vi "VectorDrive.vi"(9 "RightMotorInput":dbl, 10 "LeftMotorInput":dbl) -> (1 "RightMotorOutput":dbl, 2 "LeftMotorOutput":dbl)   [LabVIEW 2015]
uses:
  <vilib>/addons/control/pid/pid.llb/PID (DBL).vi
  navx-mxp/labview/navX Library v2/navX Library v2.lvlib
  <vilib>/addons/control/pid/NI_PID_pid.lvlib
panel:
  in  "PID gains":T1={"proportional gain (Kc)"=12.0, "integral time (Ti, min)"=0.0, "derivative time (Td, min)"=0.0015}
  in  "setpoint":dbl format="%.2f"
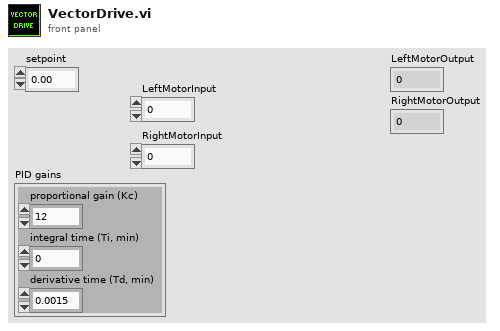
[diagram p1: front panel]
types:
  T1 = cluster{"proportional gain (Kc)":dbl, "integral time (Ti, min)":dbl, "derivative time (Td, min)":dbl}
  T2 = typedef "navX Library v2.lvlib/Z900_navX_DeviceTypeDef.ctl" = cluster{"Interface":cluster{"Protocol":T3, "Update Rate (4Hz-60Hz)":u8, "navX Open TypeDef":variant}, "Notify Packet":refnum<notifier>, "Loop VI Refnum":refnum<vi>, "Ready to Close Occurrence Refnum":refnum<k4>}
  T3 = typedef "navX Library v2.lvlib/Z900_navX_ProtocolTypeDef.ctl" = enum16{"SERIAL", "I2C", "SPI"}
  T4 = cluster{"Yaw":dbl, "Roll":dbl, "Pitch":dbl, "Heading":dbl, "Fused Heading":dbl}
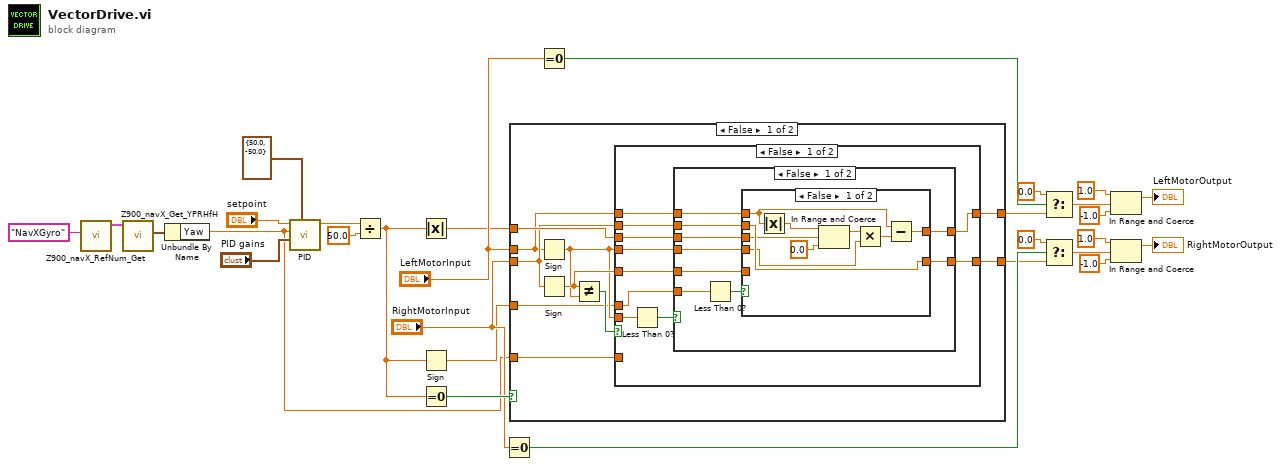
[diagram p0: block diagram]
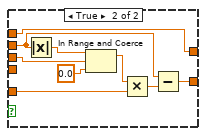
[diagram p2: hidden frame]
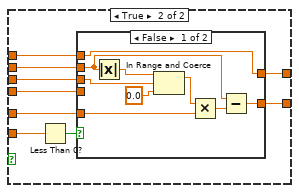
[diagram p3: hidden frame]
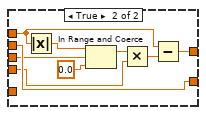
[diagram p4: hidden frame]
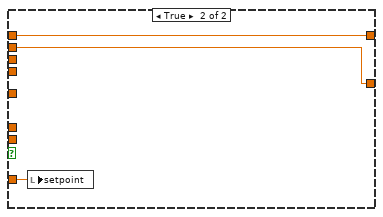
[diagram p5: hidden frame]
diagram:
  n1 = call "Z900_navX_RefNum_Get.vi"("refnum name"="NavXGyro") -> ("navX Device"=w28:T2)  [unwired: 9 in, 1 out]
  n2 = call "Z900_navX_Get_YPRHfH.vi"("navX Device"=w28) -> ("YRPHfH"=w27:T4)  [unwired: 7 in, 3 out]
  n3 = Unbundle By Name(w27) -> ("Yaw"=w12:dbl)
  n4 = call-poly <vilib>:"PID.vi"("output range"=cluster{"output high":dbl, "output low":dbl} {"output high"=50.0, "output low"=-50.0}, "PID gains"="PID gains", "process variable"=w12, "setpoint"="setpoint") -> ("output"=w1:dbl)  [unwired: 6 in, 1 out]
  n5 = Divide(x=w1, y=50.0) -> (x/y=w11:dbl)
  n6 = Absolute Value(x=w11) -> (abs(x)=w13:dbl)
  n7 = Sign(1:w11) -> (0:w10:dbl)
  n8 = Equal To 0?(x=w11) -> (x = 0?=w22:bool)
  n9 = Equal To 0?(x="RightMotorInput") -> (x = 0?=w17:bool)
  n10 = case shown="False" w22 {
    tunnel: "LeftMotorInput" -> [w34 w108]
    tunnel: "RightMotorInput" -> [w37 w107]
    tunnel: [w33 w108] -> w18
    tunnel: [w35 w107] -> w15
    tunnel: w13 -> [w38 _]
    tunnel: w12 -> [w31 _]
    tunnel: w10 -> [w30 _]
    frame False {
      n11 = Sign(1:w34) -> (0:w32:dbl)
      n12 = Sign(1:w37) -> (0:w36:dbl)
      n13 = Not Equal?(x=w36, y=w32) -> (x != y?=w39:bool)
      n14 = case shown="False" w39 {
        tunnel: w32 -> [w48 _]
        tunnel: w38 -> [w47 _]
        tunnel: w37 -> [w46 w105]
        tunnel: w36 -> [w45 _]
        tunnel: [w44 w105] -> w35
        tunnel: w34 -> [w43 w106]
        tunnel: [w42 w106] -> w33
        tunnel: w32 -> [w41 _]
        tunnel: w31 -> [_ w104]
        tunnel: w30 -> [w40 _]
        frame False {
          n15 = Less Than 0?(x=w48) -> (x < 0?=w49:bool)
          n16 = case shown="False" w49 {
            tunnel: w47 -> [w51 w80]
            tunnel: w46 -> [w55 w81]
            tunnel: w45 -> [w50 w82]
            tunnel: [w54 w77] -> w44
            tunnel: w43 -> [w53 w83]
            tunnel: [w56 w78] -> w42
            tunnel: w41 -> [w52 w79]
            tunnel: w40 -> [w58 w84]
            frame False {
              n17 = Less Than 0?(x=w58) -> (x < 0?=w57:bool)
              n18 = case shown="False" w57 {
                tunnel: [w67 w68] -> w56
                tunnel: [w66 w69] -> w54
                tunnel: w55 -> [w66 w71]
                tunnel: w53 -> [w60 w68]
                tunnel: w52 -> [w63 _]
                tunnel: w51 -> [w62 w70]
                tunnel: w50 -> [_ w72]
                frame False {
                  n19 = Absolute Value(x=w60) -> (abs(x)=w59:dbl)
                  n20 = In Range and Coerce(upper limit=w59, x=w62, lower limit=0.0) -> (coerced(x)=w64:dbl)  [unwired: 1 out]
                  n21 = Multiply(x=w64, y=w63) -> (x*y=w65:dbl)
                  n22 = Subtract(x=w60, y=w65) -> (x-y=w67:dbl)
                }
                frame True {
                  n23 = Absolute Value(x=w71) -> (abs(x)=w73:dbl)
                  n24 = In Range and Coerce(upper limit=w73, x=w70, lower limit=0.0) -> (coerced(x)=w75:dbl)  [unwired: 1 out]
                  n25 = Multiply(x=w75, y=w72) -> (x*y=w76:dbl)
                  n26 = Subtract(x=w71, y=w76) -> (x-y=w69:dbl)
                }
              }
            }
            frame True {
              n27 = Less Than 0?(x=w84) -> (x < 0?=w85:bool)
              n28 = case shown="False" w85 {
                tunnel: [w86 w103] -> w78
                tunnel: [w87 w102] -> w77
                tunnel: w81 -> [w89 w102]
                tunnel: w83 -> [w86 w96]
                tunnel: w79 -> [_ w99]
                tunnel: w80 -> [w88 w98]
                tunnel: w82 -> [w90 _]
                frame False {
                  n29 = Absolute Value(x=w89) -> (abs(x)=w91:dbl)
                  n30 = In Range and Coerce(upper limit=w91, x=w88, lower limit=0.0) -> (coerced(x)=w93:dbl)  [unwired: 1 out]
                  n31 = Multiply(x=w93, y=w90) -> (x*y=w94:dbl)
                  n32 = Subtract(x=w89, y=w94) -> (x-y=w87:dbl)
                }
                frame True {
                  n33 = Absolute Value(x=w96) -> (abs(x)=w95:dbl)
                  n34 = In Range and Coerce(upper limit=w95, x=w98, lower limit=0.0) -> (coerced(x)=w100:dbl)  [unwired: 1 out]
                  n35 = Multiply(x=w100, y=w99) -> (x*y=w101:dbl)
                  n36 = Subtract(x=w96, y=w101) -> (x-y=w103:dbl)
                }
              }
            }
          }
        }
        frame True {
          n37 = local write "setpoint"(w104) -> ()
        }
      }
    }
    frame True {
    }
  }
  n38 = Equal To 0?(x="LeftMotorInput") -> (x = 0?=w21:bool)
  n39 = Select(t=0.0, s=w21, f=w18) -> (s? t:f=w9:dbl)
  n40 = Select(t=0.0, s=w17, f=w15) -> (s? t:f=w3:dbl)
  n41 = In Range and Coerce(upper limit=1.0, x=w9, lower limit=-1.0) -> (coerced(x)=→"LeftMotorOutput":dbl)  [unwired: 1 out]
  n42 = In Range and Coerce(upper limit=1.0, x=w3, lower limit=-1.0) -> (coerced(x)=→"RightMotorOutput":dbl)  [unwired: 1 out]
